vi "Title-Remove.vi"(1 "Parameters":variant, 2 "Remove First":bool) -> (0 "Variant":variant)   [LabVIEW 2019]
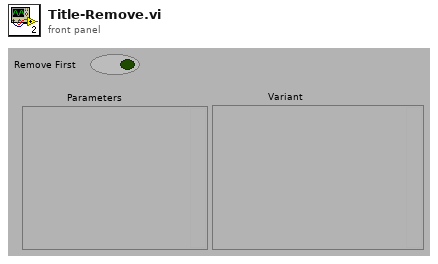
[diagram p1: front panel]
types:
  T1 = typedef "Instrument Properties.ctl" = cluster{"Public":T2, "Private":T3}
  T2 = typedef "Public.ctl" = cluster{"Column Name":string[], "Trace Color":u32[]}
  T3 = typedef "Private.ctl" = cluster{"Path":path, "VI Refnum":T4, "Name":string, "# of Values":i32, "Scale Factors":dbl[], "Display":T5[], "Offset":dbl[]}
  T4 = typedef "Instrument Ref.ctl" = refnum<vi>
  T5 = typedef "SystemCheckBox-resize.ctl" = bool
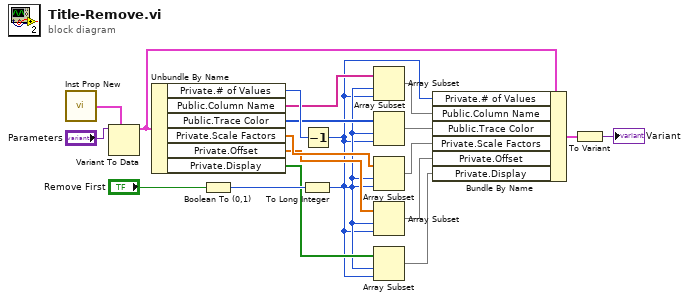
[diagram p0: block diagram]
diagram:
  n1 = call "Inst Prop New.vi"() -> ("Instrument Prop Out"=w18:T1)
  n2 = Variant To Data(type=w18, Variant="Parameters") -> (data=w16:T1)  [unwired: 1 in, 1 out]
  n3 = Unbundle By Name(w16) -> ("Private.# of Values"=w15:i32, "Public.Column Name"=w14:string[], "Public.Trace Color"=w12:u32[], "Private.Scale Factors"=w8:dbl[], "Private.Offset"=w3:dbl[], "Private.Display"=w5:T5[])
  n4 = Boolean To (0,1)(Boolean="Remove First") -> (0, 1=w9:i16)
  n5 = To Long Integer(number=w9) -> (32bit integer=w2:i32)
  n6 = Decrement(x=w15) -> (x-1=w1:i32)
  n7 = Array Subset(array=w14, index=w2, length=w1) -> (w17:string[])
  n8 = Array Subset(array=w12, index=w2, length=w1) -> (w11:u32[])
  n9 = Array Subset(array=w8, index=w2, length=w1) -> (w7:dbl[])
  n10 = Array Subset(array=w3, index=w2, length=w1) -> (w4:dbl[])
  n11 = Array Subset(array=w5, index=w2, length=w1) -> (w6:T5[])
  n12 = Bundle By Name(cluster=w16, "Private.# of Values"=w1, "Public.Column Name"=w17, "Public.Trace Color"=w11, "Private.Scale Factors"=w7, "Private.Offset"=w4, "Private.Display"=w6) -> (w13:T1)
  n13 = To Variant(anything=w13) -> (Variant=→"Variant":variant)
